vi "AMX-CCD4 自动处理图像.vi"(8 "error in (no error)":errorcluster caption="错误输入（无错误）", 9 "A/B段位置切换":bool, 10 "数值 2":i32, 11 "All Files in Dir 2":path[](array[path])) -> (0 "error out":errorcluster caption="错误输出", 1 "结果":bool, 2 "颗粒物有无判断":bool, 3 "处理时间":dbl)   [LabVIEW 2017]
uses:
  Global System.vi
panel:
  out "结果数组":bool[](array[boolean])
  out "颗粒物位置坐标":cluster{"X":dbl, "Y":dbl}[](array[cluster]) {"Y" format="%.2f"; "X" format="%.2f"}
  out "Image In":T1(plugin-control)
  out "Image Out":T1(plugin-control)
  out "颗粒物大小显示":dbl[](array[numeric])
  out "单个图片路径":path
  in  "颗粒物个数阈值":i32
  out "处理完成信号":bool
  out "子字符串":string
  out "处理完成文件":string[](array[string])
  out "All Files in Dir":path[](array[path]) caption="目录中的所有文件"
  out "未处理文件":string[](array[string])
  out "x = y?":bool[](array[boolean])
  out "数值 3":i32
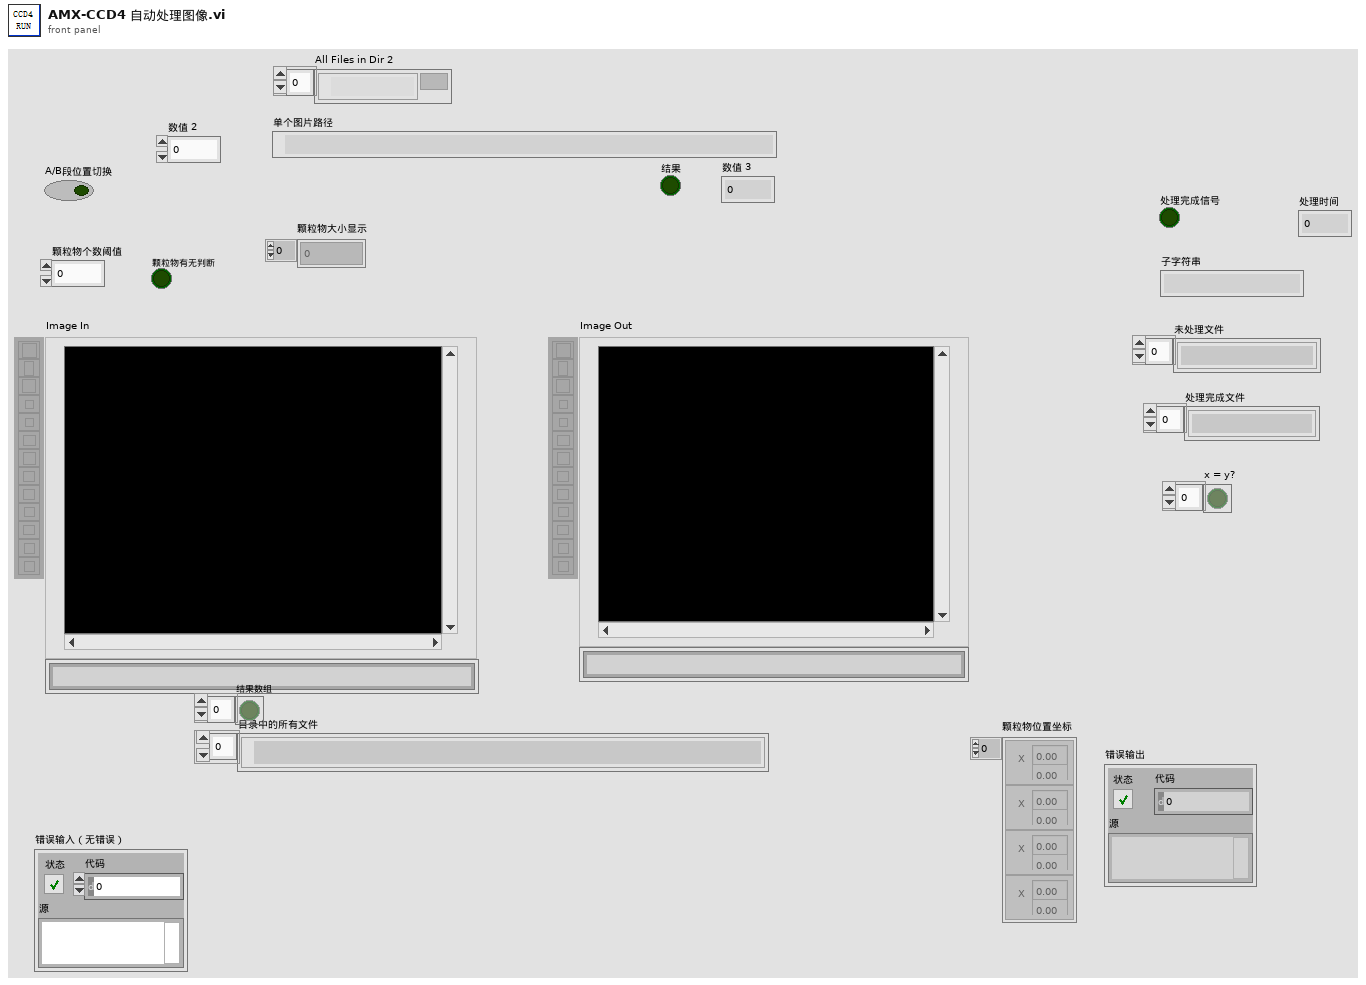
[diagram p1: front panel]
types:
  T1 = typedef "IMAQ Image.ctl" = refnum<image>
  T2 = typedef "IMAQ Rectangle" = cluster{"Left":i32, "Top":i32, "Right":i32, "Bottom":i32, "Rotation":dbl}
  T3 = cluster{"Rectangle":T2, "Threshold Limits (Threshold 1)":cluster{"Lower value":sgl, "Upper value":sgl}, "Keep/Remove Particles ":bool, "Connectivity 4/8 (8) ":bool, "Selection Values (Particle Filter 1)":cluster{"Measurement Parameter":i32, "Range Lower Value":dbl, "Range Upper Value":dbl, "Range":bool, "Measurement Type":bool}[], "Corner Options (Feature Detection 1)":cluster{"Detector type":enum32{"Harris Corner", "Shi-Tomasi Corner"}, "Kernel size":i32, "Min Corner Point Strength":dbl}, "Pyramid level (Feature Detection 1)":u32, "Method ":i32, "Look For":u32, "Method 2":i32, "ROI Descriptor (Clamp (Rake) 1)":cluster{"Global Rectangle":i32[], "Contours":cluster{"ID":enum32{"External", "Internal"}, "Type":u32, "Coordinates":i32[]}[]}}
  T4 = typedef "IMAQ Curve Parameters.ctl" = cluster{"Extraction Mode":u32, "Edge Threshold":i32, "Edge Filter Size":u32, "Min Length":i32, "Row Search Step Size":i32, "Col Search Step Size":i32, "Max Endpoint Gap":i32, "Closed":bool, "Subpixel":bool}
  T5 = cluster{"Curve Extraction Settings ":T4, "Color Mode (Histogram 1)":u16, "Range (Threshold 1)":cluster{"Lower value":sgl, "Upper value":sgl}, "Clamp Settings (Max Clamp 1)":cluster{"Angle Range (+/-)":dbl, "Edge Polarity":cluster{"Start":u32, "End":u32}}, "Settings (Clamp (Rake) 1)":cluster{"Contrast":i32, "Filter width":i32, "Steepness":i32, "Subsampling Ratio":u32, "Show Search Area":bool, "Show Search Lines":bool, "Show Edges Found":bool, "Show Result":bool}, "直径设定":cluster{"Lower value":sgl, "Upper value":sgl}}
  T6 = typedef "Image Type" = u32
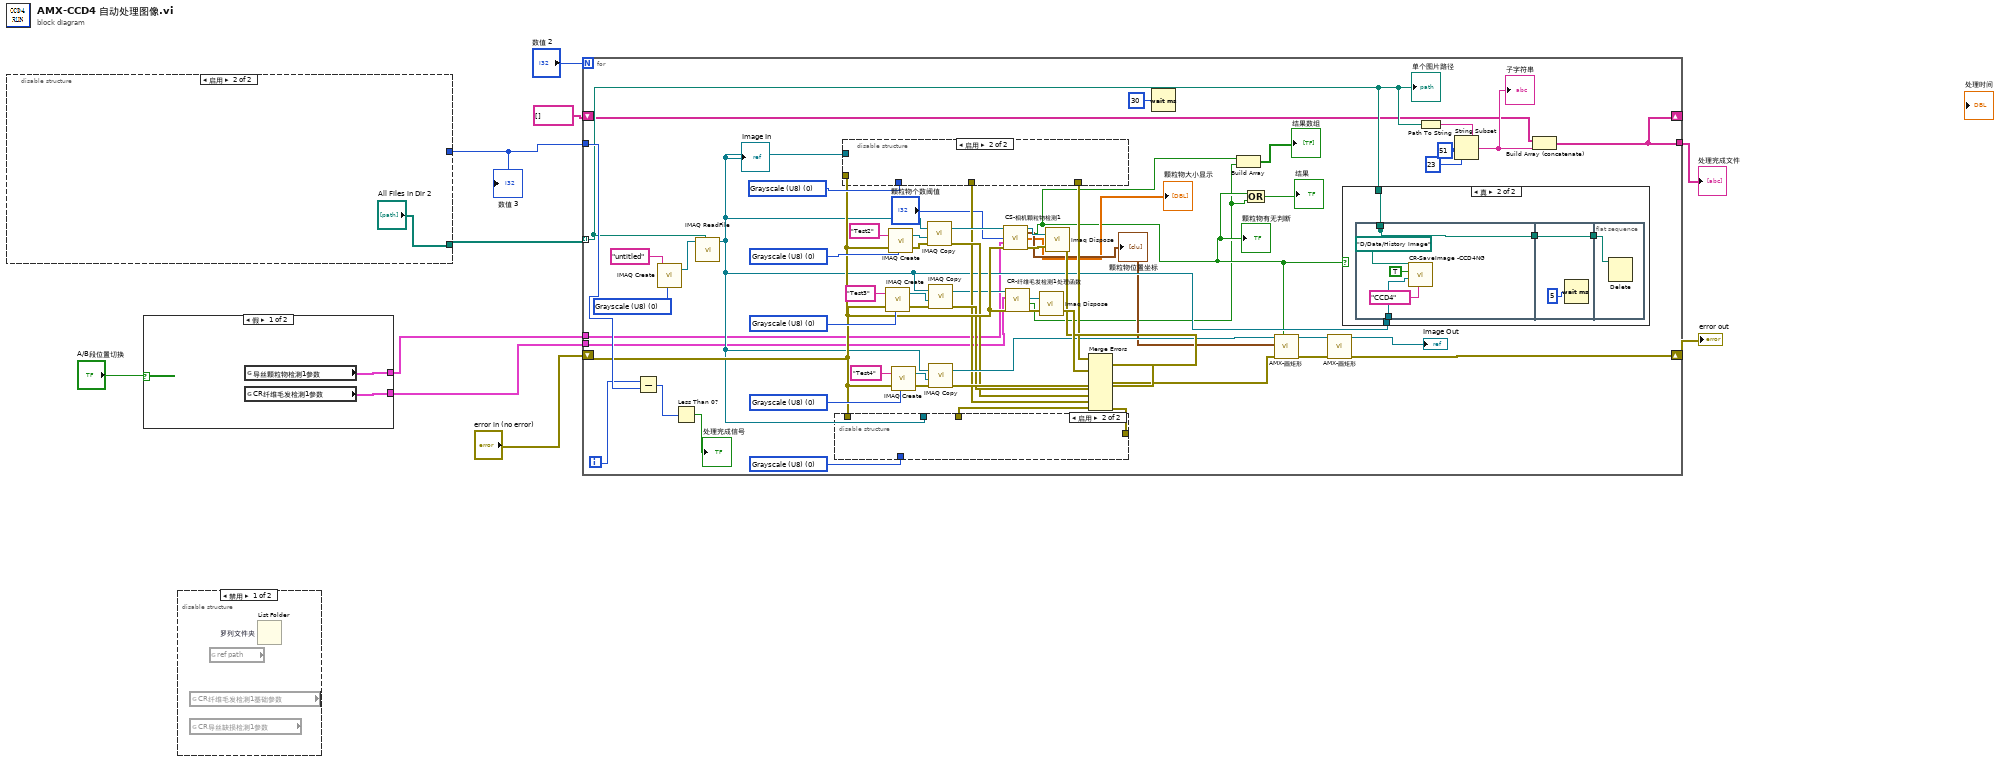
[diagram p0: block diagram]
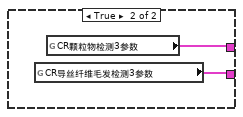
[diagram p2: hidden frame]
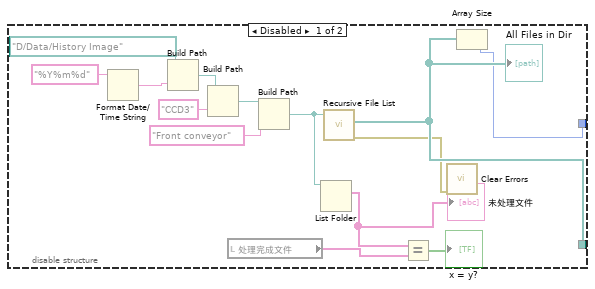
[diagram p3: hidden frame]
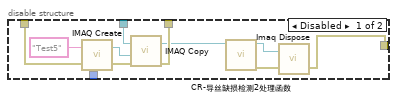
[diagram p4: hidden frame]
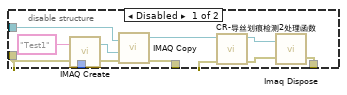
[diagram p5: hidden frame]
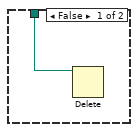
[diagram p6: hidden frame]
diagram:
  n1 = disable-structure shown="启用" {
    disable-tunnel: [w11 _] -> w1
    disable-tunnel: [w17 "All Files in Dir 2"] -> w9
    frame Disabled {
      n2 = Format Date/Time String(time format string (%c)="%Y%m%d" ("时间格式字符串(%c)")) -> (date/time string=w18:string)  [unwired: 2 in]
      n3 = Build Path(base path=path "D:/Data/History Image" ("基路径"), name or relative path=w18) -> (appended path=w21:path)
      n4 = Build Path(base path=w21, name or relative path="CCD3" ("名称或相对路径")) -> (appended path=w19:path)
      n5 = local read "处理完成文件"() -> (w14:string[])
      n6 = Build Path(base path=w19, name or relative path="Front conveyor" ("名称或相对路径")) -> (appended path=w16:path)
      n7 = List Folder(path=w16) -> (filenames=w15:string[])  [unwired: 3 in, 3 out]
      "未处理文件" <- w15
      n8 = call <vilib>:"Recursive File List.vi"("Folder Path"=w16) -> ("error out"=w12:errorcluster, "All Files in Dir"=w17:path[])  [unwired: 6 in, 3 out]
      "All Files in Dir" <- w17
      n9 = Equal?(x=w15, y=w14) -> (x = y?=→"x = y?":bool[])
      n10 = call <vilib>:"Clear Errors.vi"("error in (no error)"=w12) -> ()  [unwired: 5 in, 2 out]
      n11 = Array Size(array=w17) -> (size(s)=w11:i32)
    }
    frame Enabled {
    }
  }
  "数值 3" <- w1
  n12 = case shown="假" "A/B段位置切换" {
    tunnel: [w27 w29] -> w3
    tunnel: [w26 w28] -> w2
    frame False {
      n13 = global read "Global System.vi" "导丝颗粒物检测1参数"() -> (w27:T3)
      n14 = global read "Global System.vi" "CR纤维毛发检测1参数"() -> (w26:T5)
    }
    frame True {
      n15 = global read "Global System.vi" "CR导丝纤维毛发检测3参数"() -> (w28:T5)
      n16 = global read "Global System.vi" "CR颗粒物检测3参数"() -> (w29:T3)
    }
  }
  n17 = disable-structure shown="禁用" {
    frame Disabled {
      n18 = global read "Global System.vi" "CR纤维毛发检测1基础参数"() -> ()  [unwired: 1 out]
      n19 = global read "Global System.vi" "CR导丝缺损检测1参数"() -> ()  [unwired: 1 out]
      n20 = global read "Global System.vi" "ref path"() -> ()  [unwired: 1 out]
      n21 = List Folder "罗列文件夹"() -> ()  [unwired: 4 in, 4 out]
    }
    frame Enabled {
    }
  }
  n22 = for {
    N: "数值 2" -> [_]
    tunnel: w9 -> [w53] mode=indexing
    shift-right: [w90] -> w8
    shift-left: "error in (no error)" -> [w45]
    tunnel: w1 -> [w55]
    shift-right: [w47] -> _
    shift-left: string[] [] ("添加的数组") -> [w48]
    tunnel: [w47] -> w6
    tunnel: w3 -> [w31]
    tunnel: w2 -> [w30]
    i -> [w54]
    w59 = T6 0 items=["Grayscale (U8)", "Grayscale (I16)", "Grayscale (SGL)", "Complex (CSG)", "RGB (U32)", "HSL (U32)", "RGB (U64)", "Grayscale (U16)"] ("Image Type")
    w64 = T6 0 items=["Grayscale (U8)", "Grayscale (I16)", "Grayscale (SGL)", "Complex (CSG)", "RGB (U32)", "HSL (U32)", "RGB (U64)", "Grayscale (U16)"] ("Image Type")
    w65 = T6 0 items=["Grayscale (U8)", "Grayscale (I16)", "Grayscale (SGL)", "Complex (CSG)", "RGB (U32)", "HSL (U32)", "RGB (U64)", "Grayscale (U16)"] ("Image Type")
    w67 = T6 0 items=["Grayscale (U8)", "Grayscale (I16)", "Grayscale (SGL)", "Complex (CSG)", "RGB (U32)", "HSL (U32)", "RGB (U64)", "Grayscale (U16)"] ("Image Type")
    w75 = T6 0 items=["Grayscale (U8)", "Grayscale (I16)", "Grayscale (SGL)", "Complex (CSG)", "RGB (U32)", "HSL (U32)", "RGB (U64)", "Grayscale (U16)"] ("Image Type")
    w76 = T6 0 items=["Grayscale (U8)", "Grayscale (I16)", "Grayscale (SGL)", "Complex (CSG)", "RGB (U32)", "HSL (U32)", "RGB (U64)", "Grayscale (U16)"] ("Image Type")
    n23 = Subtract(x=w54, y=w55) -> (x-y=w57:i32)
    n24 = call "IMAQ Create"("Image Name"="untitled", "Image Type"=w76) -> ("New Image"=w78:T1)  [unwired: 3 in, 1 out]
    n25 = Less Than 0?(x=w57) -> (x < 0?=→"处理完成信号":bool)
    n26 = call "IMAQ ReadFile"("File Path"=w53, "Image"=w78) -> ("Image Out"=w40:T1)  [unwired: 5 in, 4 out]
    "Image In" <- w40
    n27 = disable-structure shown="启用" {
      disable-tunnel: [w101 _] -> w85
      disable-tunnel: w65 -> [w99 _]
      disable-tunnel: w45 -> [w95 _]
      disable-tunnel: [w94 _] -> w41
      disable-tunnel: w40 -> [w93 _]
      frame Disabled {
        n28 = call "IMAQ Create"("Image Name"="Test5", "Image Type"=w99, "error in (no error)"=w95) -> ("New Image"=w98:T1, "error out"=w97:errorcluster)  [unwired: 2 in]
        n29 = call "IMAQ Copy"("error in (no error)"=w97, "Image Dst"=w98, "Image Src"=w93) -> ("error out"=w94:errorcluster, "Image Dst Out"=w91:T1)  [unwired: 3 in]
        n30 = call "CR-导丝缺损检测2处理函数.vi"("Image in"=w91) -> ("error out"=w96:errorcluster, "Image out"=w92:T1)  [unwired: 7 in, 2 out]
        n31 = call "Imaq Dispose"("Image"=w92, "error in (no error)"=w96) -> ("error out"=w101:errorcluster)  [unwired: 4 in]
      }
      frame Enabled {
      }
    }
    n32 = disable-structure shown="启用" {
      disable-tunnel: [w112 _] -> w82
      disable-tunnel: w59 -> [w111 _]
      disable-tunnel: w45 -> [w106 _]
      disable-tunnel: [w105 _] -> w42
      disable-tunnel: w40 -> [w104 _]
      frame Disabled {
        n33 = call "IMAQ Create"("Image Name"="Test1", "Image Type"=w111, "error in (no error)"=w106) -> ("New Image"=w108:T1, "error out"=w109:errorcluster)  [unwired: 2 in]
        n34 = call "IMAQ Copy"("error in (no error)"=w109, "Image Dst"=w108, "Image Src"=w104) -> ("error out"=w105:errorcluster, "Image Dst Out"=w103:T1)  [unwired: 3 in]
        n35 = call "CR-导丝划痕检测2处理函数.vi"("error in (no error)"=w106, "Image in"=w103) -> ("error out"=w110:errorcluster, "Image out"=w102:T1)  [unwired: 6 in, 2 out]
        n36 = call "Imaq Dispose"("Image"=w102, "error in (no error)"=w110) -> ("error out"=w112:errorcluster)  [unwired: 4 in]
      }
      frame Enabled {
      }
    }
    n37 = call "IMAQ Create"("Image Name"="Test3", "Image Type"=w64, "error in (no error)"=w45) -> ("New Image"=w61:T1, "error out"=w60:errorcluster)  [unwired: 2 in]
    n38 = call "IMAQ Create"("Image Name"="Test2", "Image Type"=w75, "error in (no error)"=w45) -> ("New Image"=w71:T1, "error out"=w70:errorcluster)  [unwired: 2 in]
    n39 = call "IMAQ Create"("Image Name"="Test4", "Image Type"=w67, "error in (no error)"=w45) -> ("New Image"=w68:T1, "error out"=w69:errorcluster)  [unwired: 2 in]
    n40 = call "IMAQ Copy"("error in (no error)"=w70, "Image Dst"=w71, "Image Src"=w40) -> ("error out"=w43:errorcluster, "Image Dst Out"=w46:T1)  [unwired: 3 in]
    n41 = call "IMAQ Copy"("error in (no error)"=w60, "Image Dst"=w61, "Image Src"=w40) -> ("error out"=w44:errorcluster, "Image Dst Out"=w36:T1)  [unwired: 3 in]
    n42 = call "IMAQ Copy"("error in (no error)"=w69, "Image Dst"=w68, "Image Src"=w40) -> ("error out"=w87:errorcluster, "Image Dst Out"=w80:T1)  [unwired: 3 in]
    n43 = call "CS-相机颗粒物检测1.vi"("Image in"=w46, "颗粒物个数阈值"="颗粒物个数阈值", "导丝颗粒物检测1参数"=w31, "error in (no error)"=w45) -> ("颗粒物位置坐标"=w38:cluster{"X":dbl, "Y":dbl}[], "Image out"=w74:T1, "颗粒物有无显示"=w33:bool, "颗粒物大小显示"=→"颗粒物大小显示":dbl[], "error out"=w73:errorcluster)  [unwired: 5 in, 2 out]
    "颗粒物有无判断" <- w33
    "颗粒物位置坐标" <- w38
    n44 = call "CR-纤维毛发检测1处理函数.vi"("error in (no error)"=w45, "UI电源线正面漏线参数"=w30, "Image in"=w36) -> ("error out"=w63:errorcluster, "纤维毛发"=w32:bool, "Image out"=w35:T1)  [unwired: 4 in, 2 out]
    n45 = call "Imaq Dispose"("Image"=w35, "error in (no error)"=w63) -> ("error out"=w84:errorcluster)  [unwired: 4 in]
    n46 = call "Imaq Dispose"("Image"=w74, "error in (no error)"=w73) -> ("error out"=w83:errorcluster)  [unwired: 4 in]
    n47 = Merge Errors(w82, w83, w84, w87, w85, w44, w43, w42, w41) -> (w81:errorcluster)
    n48 = Wait (ms)(milliseconds to wait=u32 30 ("等待时间（毫秒）")) -> ()  [unwired: 1 out]
    n49 = Build Array(w33, w32) -> (→"结果数组":bool[])
    n50 = Or(x=w33, y=w32) -> (x .or. y?=→"结果":bool)
    n51 = call "AMX-画矩形.vi"("布尔"=w33, "error in (no error)"=w81, "颗粒物位置坐标"=w38, "Image In"=w80) -> ("error out"=w88:errorcluster, "Image Out"=w89:T1)  [unwired: 6 in]
    n52 = call "AMX-画矩形.vi"("error in (no error)"=w88, "Image In"=w89) -> ("error out"=w90:errorcluster, "Image Out"=→"Image Out":T1)  [unwired: 8 in]
    n53 = case shown="真" w33 {
      tunnel: w53 -> [w113 w116]
      tunnel: w40 -> [_ w117]
      frame False {
        n54 = Delete(path (use dialog)=w113) -> ()  [unwired: 4 in, 3 out]
      }
      frame True {
        n55 = flat-sequence {
          tunnel: w117 -> [w122]
          tunnel: [w118] -> _
          tunnel: w116 -> [w118]
          tunnel: [w118] -> w115
          tunnel: w115 -> [w123]
          tunnel: [w123] -> w114
          tunnel: w114 -> [w125]
          frame #0 {
            n56 = call "CR-SaveImage -CCD4NG.vi"("CCD Name"="CCD4", "Image in"=w122, "布尔"=TRUE, "基路径"=path "D:/Data/History Image") -> ()  [unwired: 7 in, 1 out]
          }
          frame #1 {
            n57 = Wait (ms)(milliseconds to wait=u32 5 ("等待时间（毫秒）")) -> ()  [unwired: 1 out]
          }
          frame #2 {
            n58 = Delete(path (use dialog)=w125) -> ()  [unwired: 4 in, 3 out]
          }
        }
      }
    }
    n59 = Path To String(path=w53) -> (string=w52:string)
    n60 = String Subset(string=w52, offset (0)=51 ("偏移量(0)"), length (rest)=23 ("长度（剩余）")) -> (substring=w49:string)
    "子字符串" <- w49
    n61 = Build Array (concatenate)(w48, w49) -> (w47:string[])
    "单个图片路径" <- w53
  }
  "error out" <- w8
  "处理完成文件" <- w6
